vi "Get-active-motors.vi"(8 "error in (no error)":errorcluster, 11 "Available motors in":refnum<class "Motor-assembly.lvclass">) -> (0 "error out":errorcluster, 2 "Active motors":refnum<class "Motor.lvclass">[](array[class]), 3 "Available motors out":refnum<class "Motor-assembly.lvclass">)   [LabVIEW 2013, in "PowderDeposition.lvlib" / "Motor-assembly.lvclass"]
uses:
  Motor-assembly.lvclass
  Motor/Motor.lvclass
  Motor-assembly.lvclass/Motor-assembly.ctl
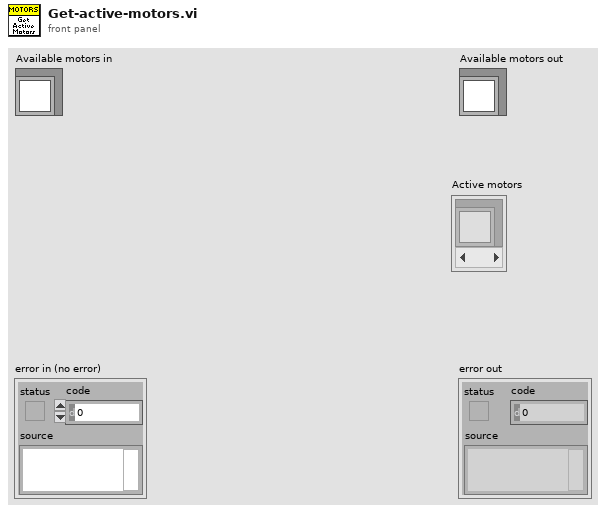
[diagram p1: front panel]
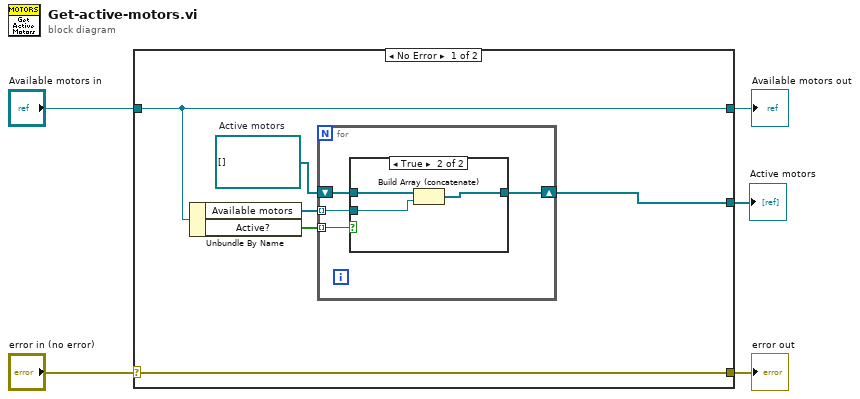
[diagram p0: block diagram]
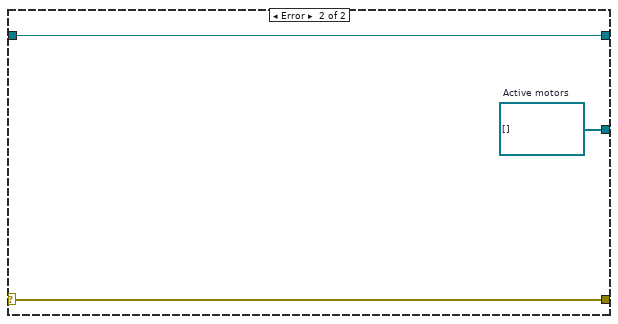
[diagram p3: hidden frame]
diagram:
  n1 = case shown="No Error" "error in (no error)" {
    selector: "error in (no error)" -> [w11 w22]
    tunnel: [w11 w22] -> w4
    tunnel: [w10 w21] -> w2
    tunnel: "Available motors in" -> [w10 w21]
    tunnel: [w6 w20] -> w1
    frame No Error {
      w7 = refnum<class "Motor.lvclass">[] []  # Active motors
      n2 = Unbundle By Name(w10) -> ("Available motors"=w9:refnum<class "Motor.lvclass">[], "Active?"=w8:bool[])
      n3 = for {
        tunnel: w9 -> [w12] mode=indexing
        tunnel: w8 -> [w15] mode=indexing
        shift-right: [w13] -> w6
        shift-left: w7 -> [w14]
        n4 = case shown="True" w15 {
          tunnel: w14 -> [w16 w19]
          tunnel: [w16 w18] -> w13
          tunnel: w12 -> [_ w17]
          frame False {
          }
          frame True {
            n5 = Build Array (concatenate)(w19, w17) -> (w18:refnum<class "Motor.lvclass">[])
          }
        }
      }
    }
    frame Error {
      w20 = refnum<class "Motor.lvclass">[] []  # Active motors
    }
  }
  "error out" <- w4
  "Available motors out" <- w2
  "Active motors" <- w1
